vi "Scaling.vi"   [LabVIEW 2014, in "NI_EP_Power Quality.lvlib"]
doc: "Scales waveforms based on the sensitivity of the voltage/current transformer or transducer. You must manually select the polymorphic instance you want to use.\n\nThis VI supports measuring single-line and multiple-line systems."
uses:
  <vilib>/addons/Electrical Power/PQ/NI_EP_Power Quality.lvlib
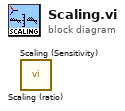
[diagram p0: block diagram]
diagram:
  n1 = call <vilib>:"Scaling (ratio).vi"() -> ()  [unwired: 13 in, 3 out]
  n2 = call <vilib>:"Scaling (Sensitivity).vi"() -> ()  [unwired: 13 in, 3 out]
